vi "OE1022D_Configure Channel Out.vi"(7 "OE1022D_Configure Channel Out":T1={"CH1 Speed"=0, "CH2 Offset(%)"=0.0, "CH1 Offset(%)"=0.0, "CH2 Expand"=1.0, "CH1 Expand"=1.0, "CH1"=0, "CH2"=0, "AUX OUT1"=1.0, "AUX OUT2"=1.0, "CH2 Speed"=0} {"CH2 Speed" items=["Slow", "Fast"]; "AUX OUT2" min=-10.0 max=10.0 format="%#.3g"; "AUX OUT1" min=-10.0 max=10.0 format="%#.3g"; "CH2" items=["A-R", "A-X", "A-Y", "A-Theta", "A-Rh1", "A-Xh1", "A-Yh1", "A-Theta h1", "A-Rh2", "A-Xh2", "A-Yh2", "A-Theta h2", "A-Noise", "A-E1", "A-E2", "A-E3", "A-E4", "B-R", "B-X", "B-Y", "B-Theta", "B-Rh1", "B-Xh1", "B-Yh1", "B-Theta h1", "B-Rh2", "B-Xh2", "B-Yh2", "B-Theta h2", "B-Noise", "B-E1", "B-E2", "B-E3", "B-E4", "AUX OUT"]; "CH1" items=["A-R", "A-X", "A-Y", "A-Theta", "A-Rh1", "A-Xh1", "A-Yh1", "A-Theta h1", "A-Rh2", "A-Xh2", "A-Yh2", "A-Theta h2", "A-Noise", "A-E1", "A-E2", "A-E3", "A-E4", "B-R", "B-X", "B-Y", "B-Theta", "B-Rh1", "B-Xh1", "B-Yh1", "B-Theta h1", "B-Rh2", "B-Xh2", "B-Yh2", "B-Theta h2", "B-Noise", "B-E1", "B-E2", "B-E3", "B-E4", "AUX OUT"]; "CH1 Expand" min=1.0 max=256.0 format="%#_3g"; "CH2 Expand" min=1.0 max=256.0 format="%#_3g"; "CH1 Offset(%)" min=-100.0 max=100.0 format="%#_5g"; "CH2 Offset(%)" min=-100.0 max=100.0 format="%#_5g"; "CH1 Speed" items=["Slow", "Fast"]}, 8 "Error in (no error)":errorcluster caption="error out（no error）", 9 "Remote Mode":u16(ring) items=["USB", "RS232", "GPIB"], 11 "VISA resource name":refnum<visa-resource-name>) -> (0 "Error out":errorcluster caption="error out", 1 "Output String":string, 3 "VISA resource  out":refnum<visa-resource-name>)   [LabVIEW 2011]
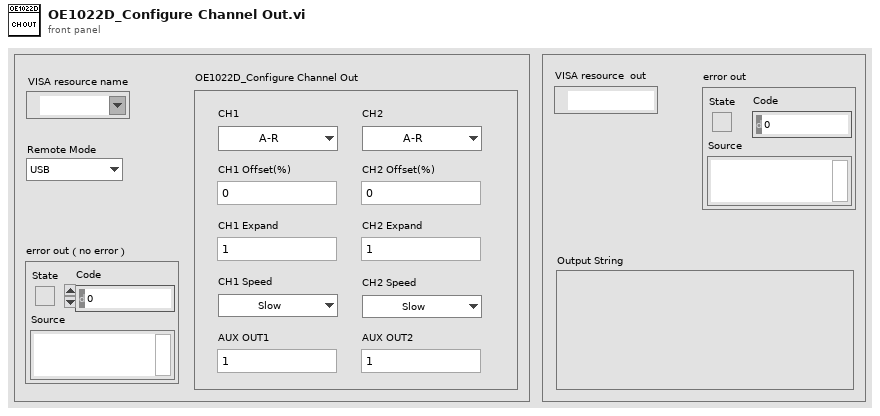
[diagram p1: front panel]
types:
  T1 = cluster{"CH1 Speed":u16, "CH2 Offset(%)":dbl, "CH1 Offset(%)":dbl, "CH2 Expand":dbl, "CH1 Expand":dbl, "CH1":u16, "CH2":u16, "AUX OUT1":dbl, "AUX OUT2":dbl, "CH2 Speed":u16}
  T2 = enum16{"ISRC", "IGND", "ICPL", "ILIN", "PHAS", "FMOD", "RSLP", "FREQ", "SWPT", "SLLM", "SULM", "SSLL", "SSLG", "STLM", "SWRM", "IRNG", "SENS", "RMOD", "OFLT", "OFSL", "SYNC", "DMOD", "HARM", "DARB", "SWVT", "SLVL", "SVLL", "SVUL", "SVSL", "SVSG", "SVTM", "SVRM", "RALL", "SNAP", "OUTP", "OAUX", "COUT", "CAUX", "COFP", "CEXP", "FPOP", "OEXP", "*IDN", "*RST", "OVLD", "INOV", "GNOV", "*PLL", "SSET", "RSET", "AGAN", "APHS", "ARSV", "ASCL", "EQCD", "EQCS", "SPED", "SRAT", "SLEN", "SSLE", "STRG", "SPRM", "STRD", "PAUS", "REST", "SPTS", "TRCA", "TEMP", "RSTU", "IHNZ", "DEQU", "SADD", "ARNG", "CSPE", "ISRCD", "IGNDD", "ICPLD", "ILIND", "PHASD", "FMODD", "RSLPD", "FREQD", "SWPTD", "SLLMD", "SULMD", "SSLLD", "SSLGD", "STLMD", "SWRMD", "SENSD", "RMODD", "OFLTD", "OFSLD", "SYNCD", "HARMD", "EQCDD", "EQCSD", "SNAPD", "OUTPD", "SWVTD", "SLVLD", "SVLLD", "SVULD", "SVSLD", "SVSGD", "SVTMD", "SVRMD", "SVDCD", "ARSVD", "AGAND", "APHSD", "ASCLD", "FPOPD", "CAUXD", "OEXPD", "SPEDD", "SRATD", "SLEND", "SSLED", "STRGD", "SPRMD", "STRDD", "PAUSD", "RESTD", "SPTSD", "TRCAD", "*IDND", "*RSTD", "INOVD", "GNOVD", "*PLLD", "SSETD", "RSETD"}
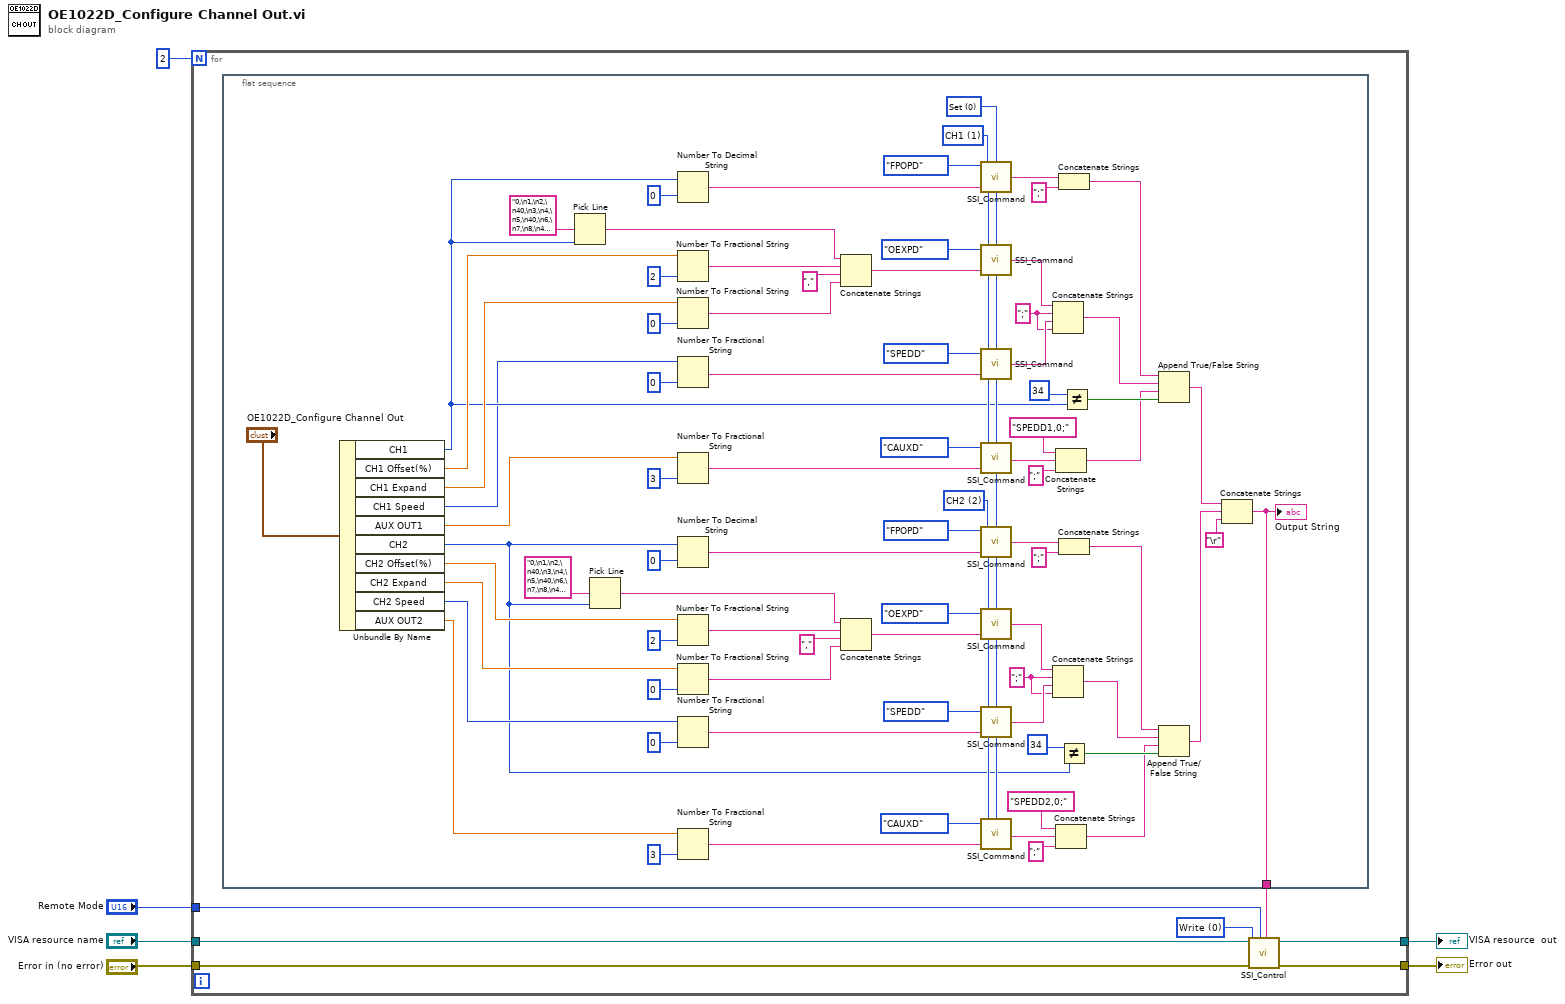
[diagram p0: block diagram]
diagram:
  n1 = for {
    N: 2 -> [_]
    tunnel: "VISA resource name" -> [w13]
    tunnel: "Remote Mode" -> [w11]
    tunnel: "Error in (no error)" -> [w10]
    tunnel: [w9] -> w3
    tunnel: [w8] -> w2
    w12 = u16 0 items=["Write", "Read"] ("Control")
    n2 = flat-sequence {
      tunnel: [w33] -> w7
      frame #0 {
        w25 = u16 2 items=["CH1"=1, "CH2"=2]
        w26 = u16 1 items=["CH1"=1, "CH2"=2]
        w44 = ";" ("替换字符串(\"\")")
        w69 = ";" ("替换字符串(\"\")")
        w29 = u16 0 items=["Set", "Query"] ("Opera")
        n3 = Unbundle By Name("OE1022D_Configure Channel Out") -> ("CH1"=w21:u16, "CH1 Offset(%)"=w76:dbl, "CH1 Expand"=w75:dbl, "CH1 Speed"=w14:u16, "AUX OUT1"=w74:dbl, "CH2"=w19:u16, "CH2 Offset(%)"=w35:dbl, "CH2 Expand"=w36:dbl, "CH2 Speed"=w37:u16, "AUX OUT2"=w38:dbl)
        n4 = Pick Line(multi-line string="0,\n1,\n2,\n40,\n3,\n4,\n5,\n40,\n6,\n7,\n8,\n40,\n9,\n40,\n40,\n40,\n40,\n10,\n11,\n12,\n40,\n13,\n14,\n15,\n40,\n16,\n17,\n18,\n40,\n19,\n40,\n40,\n40,\n40," ("多行字符串"), line index=w21) -> (output string=w17:string)  [unwired: 1 in]
        n5 = Pick Line(multi-line string="0,\n1,\n2,\n40,\n3,\n4,\n5,\n40,\n6,\n7,\n8,\n40,\n9,\n40,\n40,\n40,\n40,\n10,\n11,\n12,\n40,\n13,\n14,\n15,\n40,\n16,\n17,\n18,\n40,\n19,\n40,\n40,\n40,\n40," ("多行字符串"), line index=w19) -> (output string=w18:string)  [unwired: 1 in]
        n6 = Number To Decimal String(number=w21, width (-)=i16 0 ("精度(6)")) -> (decimal integer string=w23:string)
        n7 = Number To Fractional String(number=w76, precision (6)=i16 2 ("精度(6)")) -> (F-format string=w87:string)  [unwired: 2 in]
        n8 = Number To Fractional String(number=w75, precision (6)=i16 0 ("精度(6)")) -> (F-format string=w85:string)  [unwired: 2 in]
        n9 = Number To Fractional String(number=w14, precision (6)=i16 0 ("精度(6)")) -> (F-format string=w24:string)  [unwired: 2 in]
        n10 = Number To Fractional String(number=w74, precision (6)=i16 3 ("精度(6)")) -> (F-format string=w31:string)  [unwired: 2 in]
        n11 = Number To Decimal String(number=w19, width (-)=i16 0 ("精度(6)")) -> (decimal integer string=w28:string)
        n12 = Number To Fractional String(number=w35, precision (6)=i16 2 ("精度(6)")) -> (F-format string=w57:string)  [unwired: 2 in]
        n13 = Number To Fractional String(number=w36, precision (6)=i16 0 ("精度(6)")) -> (F-format string=w55:string)  [unwired: 2 in]
        n14 = Number To Fractional String(number=w37, precision (6)=i16 0 ("精度(6)")) -> (F-format string=w27:string)  [unwired: 2 in]
        n15 = Number To Fractional String(number=w38, precision (6)=i16 3 ("精度(6)")) -> (F-format string=w30:string)  [unwired: 2 in]
        n16 = Concatenate Strings(w17, w87, ",", w85) -> (w84:string)
        n17 = Concatenate Strings(w18, w57, ",", w55) -> (w54:string)
        n18 = call "SSI_Command.vi"("Opera"=w29, "Paramter"=w23, "channel"=w26, "Command Type"=T2."FPOPD") -> ("Output string"=w66:string)
        n19 = call "SSI_Command.vi"("Opera"=w29, "Paramter"=w84, "channel"=w26, "Command Type"=T2."OEXPD") -> ("Output string"=w90:string)
        n20 = call "SSI_Command.vi"("Opera"=w29, "Paramter"=w24, "channel"=w26, "Command Type"=T2."SPEDD") -> ("Output string"=w70:string)
        n21 = call "SSI_Command.vi"("Opera"=w29, "Paramter"=w31, "channel"=w26, "Command Type"=T2."CAUXD") -> ("Output string"=w78:string)
        n22 = call "SSI_Command.vi"("Opera"=w29, "Paramter"=w28, "channel"=w25, "Command Type"=T2."FPOPD") -> ("Output string"=w41:string)
        n23 = call "SSI_Command.vi"("Opera"=w29, "Paramter"=w54, "channel"=w25, "Command Type"=T2."OEXPD") -> ("Output string"=w59:string)
        n24 = call "SSI_Command.vi"("Opera"=w29, "Paramter"=w27, "channel"=w25, "Command Type"=T2."SPEDD") -> ("Output string"=w45:string)
        n25 = call "SSI_Command.vi"("Opera"=w29, "Paramter"=w30, "channel"=w25, "Command Type"=T2."CAUXD") -> ("Output string"=w49:string)
        n26 = Concatenate Strings(w90, w69, w70, w69) -> (w68:string)
        n27 = Concatenate Strings(w59, w44, w45, w44) -> (w43:string)
        n28 = Concatenate Strings("SPEDD1,0;" ("字符串"), w78, ";" ("替换字符串(\"\")")) -> (w71:string)
        n29 = Concatenate Strings("SPEDD2,0;" ("字符串"), w49, ";" ("替换字符串(\"\")")) -> (w46:string)
        n30 = Concatenate Strings(w66, ";" ("替换字符串(\"\")")) -> (w65:string)
        n31 = Concatenate Strings(w41, ";" ("替换字符串(\"\")")) -> (w40:string)
        n32 = Not Equal?(x=u16 34, y=w19) -> (x != y?=w47:bool)
        n33 = Not Equal?(x=u16 34, y=w21) -> (x != y?=w73:bool)
        n34 = Append True/False String(1:w73, 2:w71, 3:w68, 4:w65) -> (0:w64:string)
        n35 = Append True/False String(1:w47, 2:w46, 3:w43, 4:w40) -> (0:w39:string)
        n36 = Concatenate Strings(w64, w39, "\r") -> (w33:string)
        "Output String" <- w33
      }
    }
    n37 = call "SSI_Control.vi"("Write Buffer"=w7, "Remote Mode"=w11, "Error in (no error)"=w10, "Control"=w12, "VISA resource name"=w13) -> ("Error out"=w9:errorcluster, "VISA resource  out"=w8:refnum<visa-resource-name>)  [unwired: 3 in, 2 out]
  }
  "Error out" <- w3
  "VISA resource  out" <- w2
